vi "R Place.vi"() -> ()   [LabVIEW 2025]
panel:
  in  "Color Array":u32[][](array[colorbox])
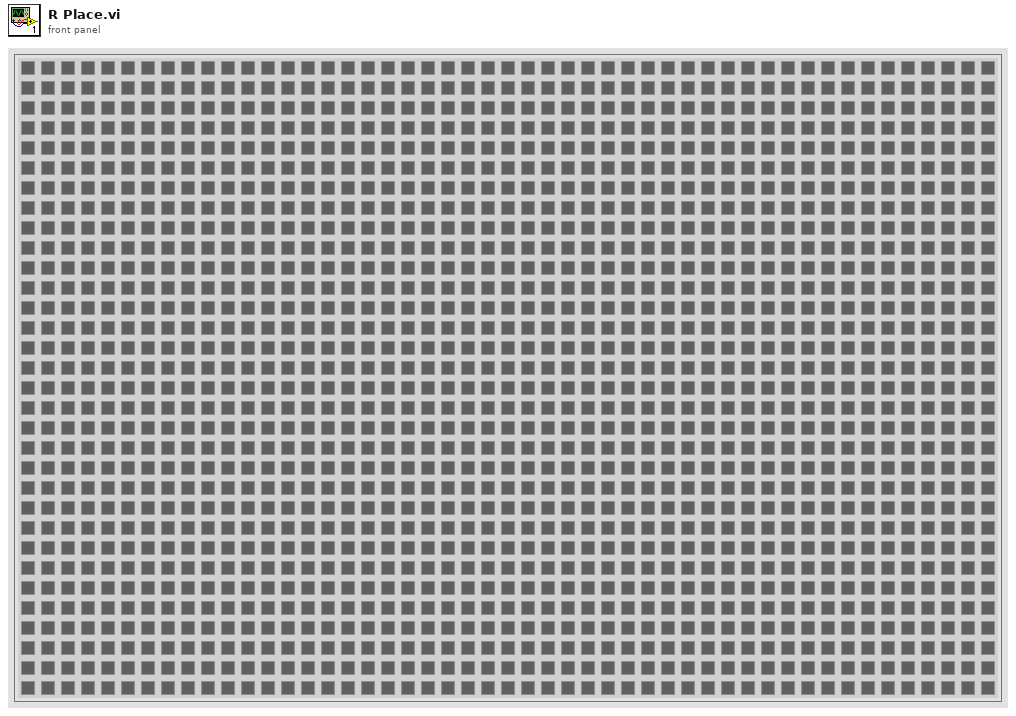
[diagram p1: front panel]
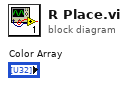
[diagram p0: block diagram]
diagram:
